vi "Calibrate.vi"(8 "error in (no error)":errorcluster, 11 "KUKA youBot arm motor_EtherCAT in":refnum<class "NI_Robotics_KUKA youBot Arm Motor_EtherCAT.lvclass">) -> (0 "error out":errorcluster, 3 "KUKA youBot arm motor_EtherCAT out":refnum<class "NI_Robotics_KUKA youBot Arm Motor_EtherCAT.lvclass">)   [LabVIEW 2017, in "NI_Robotics_KUKA youBot Host.lvlib" / "NI_Robotics_KUKA youBot Arm Motor_EtherCAT.lvclass"]
uses:
  <vilib>/robotics/KUKA youBot/Motor/Arm Motor EtherCAT/NI_Robotics_KUKA youBot Arm Motor_EtherCAT.lvclass
  <vilib>/robotics/KUKA youBot/Motor/Arm Motor EtherCAT/NI_Robotics_KUKA youBot Arm Motor_EtherCAT.lvclass/NI_Robotics_KUKA youBot Arm Motor_EtherCAT.ctl
  <vilib>/robotics/KUKA youBot/EtherCAT/EtherCAT Command.ctl
  <vilib>/robotics/KUKA youBot/EtherCAT/CmdCtrls/Param Cmd.ctl
  <vilib>/Platform/TimedLoop/XDataNode/timing_clust.ctl
  <vilib>/Platform/TimedLoop/XDataNode/nitl_modes.ctl
  <vilib>/Platform/TimedLoop/XDataNode/wakeup.ctl
  <vilib>/Platform/TimedLoop/XDataNode/XDataNode.xnode
  <vilib>/robotics/KUKA youBot/NI_Robotics_KUKA youBot Host.lvlib
  <vilib>/Platform/TimedLoop/XDataNode/XDNodeRunTimeDep.lvlib
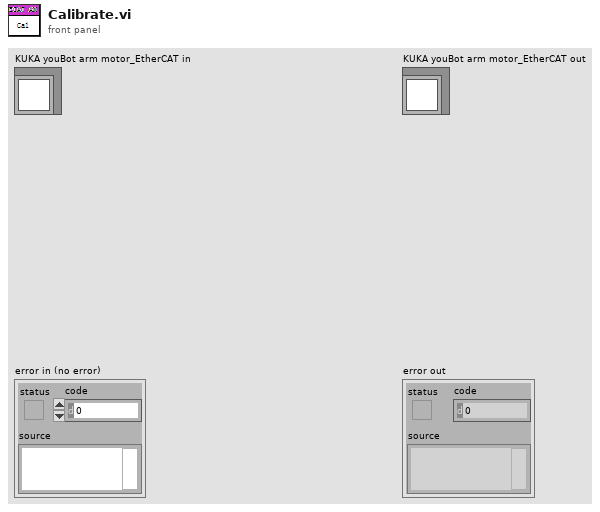
[diagram p1: front panel]
types:
  T1 = typedef "NI_Robotics_KUKA youBot Host.lvlib/EtherCAT Command.ctl" = cluster{"Module":u8, "Cmd":T2, "Type":u8, "Bank":u8, "Val":u32}
  T2 = typedef "NI_Robotics_KUKA youBot Host.lvlib/Param Cmd.ctl" = u8
  T3 = typedef "XDNodeRunTimeDep.lvlib/timing_clust.ctl" = cluster{"Expected End [f-1]":u64, "Actual End [f-1]":u64, "Finished Late? [f-1]":bool, "Expected End [i-1]":u64, "Actual End [i-1]":u64, "Finished Late? [i-1]":bool, "Expected Start [i]":u64, "Actual Start [i]":u64, "Expected Start [f]":u64, "Actual Start [f]":u64, "Source Name":string, "Structure Name":string, "Period":i64, "Deadline":i64, "Offset":i64, "Start":i64, "Priority":i32, "Timeout":i32, "Mode":T4, "Wakeup Reason":T5, "Error":errorcluster, "Source Type":string, "Secondary Source Type":string, "Global End Time":u64, "Global Start Time":u64, "Frame Duration":u64, "Iteration Duration":u64, "Assigned CPU":i32, "I/O Scan Engine Mode":u32}
  T4 = typedef "XDNodeRunTimeDep.lvlib/nitl_modes.ctl" = enum32{"No Change", "Process missed periods, maintain original phase", "Discard missed periods, maintain original phase", "Process missed periods, ignore original phase", "Discard missed periods, ignore original phase"}
  T5 = typedef "XDNodeRunTimeDep.lvlib/wakeup.ctl" = enum32{"Normal", "Aborted", "Asynchronous wakeup", "Timing source error", "Timed loop error", "Timeout"}
  T6 = typedef "NI_Robotics_KUKA youBot Host.lvlib/Mater Handler.ctl" = i32
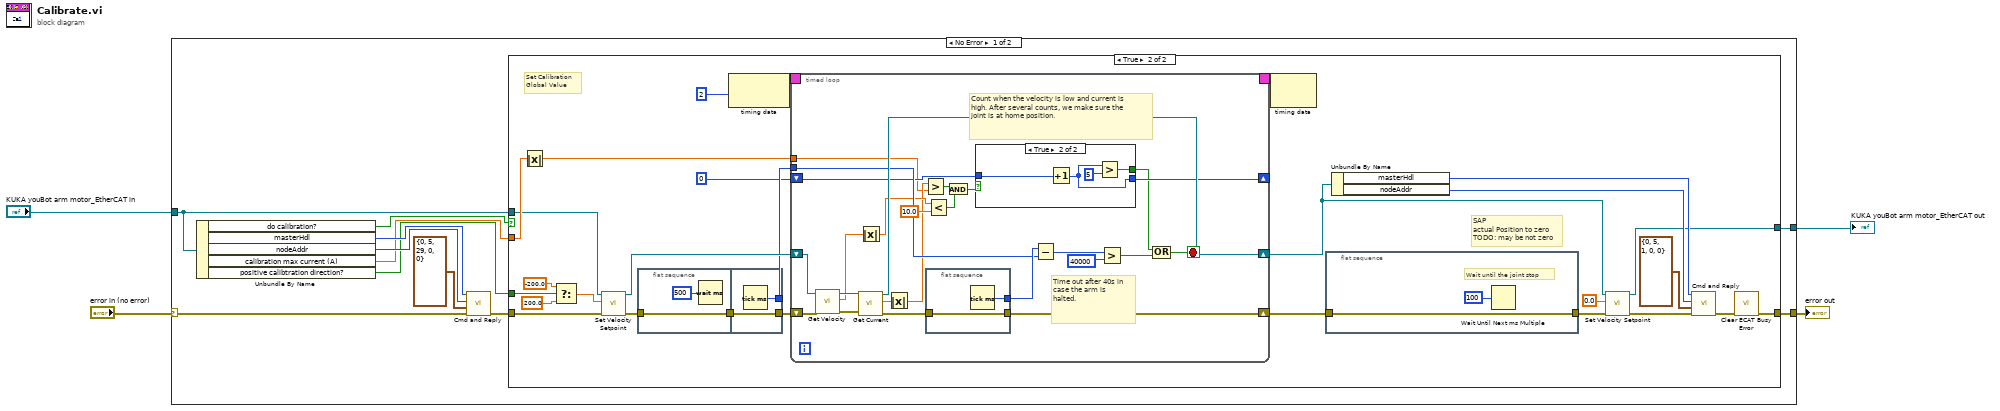
[diagram p0: block diagram]
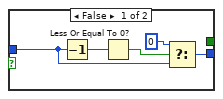
[diagram p3: hidden frame]
diagram:
  n1 = case shown="No Error" "error in (no error)" {
    selector: "error in (no error)" -> [w6 w95]
    tunnel: "KUKA youBot arm motor_EtherCAT in" -> [w7 w94]
    tunnel: [w10 w95] -> w2
    tunnel: [w9 w94] -> w1
    frame No Error {
      n2 = Unbundle By Name(w7) -> ("do calibration?"=w8:bool, "masterHdl"=w15:T6, "nodeAddr"=w14:u16, "calibration max current (A)"=w11:dbl, "positive calibtration direction?"=w12:bool)
      n3 = call <vilib>:"Cmd and Reply.vi"("error in (no error)"=w6, "EtherCAT command"=T1 {"Module"=0, "Cmd"=5, "Type"=29, "Bank"=0, "Val"=0} ("EtherCAT Command"), "nodeAddr in"=w14, "masterHdl in"=w15) -> ("error out"=w5:errorcluster)  [unwired: 3 in, 4 out]
      n4 = case shown="True" w8 {
        tunnel: w12 -> [_ w45]
        tunnel: w7 -> [w16 w26]
        tunnel: w5 -> [w17 w40]
        tunnel: w11 -> [_ w38]
        tunnel: [w17 w19] -> w10
        tunnel: [w16 w22] -> w9
        frame False {
        }
        frame True {
          # "Set Calibration\nGlobal Value"
          # "SAP\nactual Position to zero\nTODO: may be not zero"
          n5 = Absolute Value(x=w38) -> (abs(x)=w37:dbl)
          n6 = Select(t=-200.0, s=w45, f=200.0) -> (s? t:f=w31:dbl)
          n7 = call-dynamic "Set Velocity Setpoint.vi"("error in (no error)"=w40, "CCW velocity (rpm)"=w31, "KUKA youBot arm motor_EtherCAT in"=w26) -> ("error out"=w30:errorcluster, "KUKA youBot arm motor_EtherCAT out"=w39:refnum<class "NI_Robotics_KUKA youBot Arm Motor_EtherCAT.lvclass">)  [unwired: 7 in]
          n8 = flat-sequence {
            tunnel: w30 -> [w47]
            tunnel: [w47] -> w18
            tunnel: [w49] -> w29
            tunnel: [w48] -> w28
            tunnel: w18 -> [w49]
            frame #0 {
              n9 = Wait (ms)(milliseconds to wait=u32 500) -> ()  [unwired: 1 out]
            }
            frame #1 {
              n10 = Tick Count (ms)() -> (millisecond timer value=w48:u32)
            }
          }
          n11 = node-c288(i64 2 ("Period")) -> (w42:T3)
          n12 = timed-loop {
            timing: w42 -> [_]
            timing-out: [_] -> w41
            shift-right: [w76] -> w33
            shift-left: w39 -> [w61]
            tunnel: w37 -> [w52]
            shift-right: [w73] -> w36
            shift-left: w29 -> [w63]
            tunnel: w28 -> [w71]
            shift-right: [w66] -> _
            shift-left: 0 -> [w67]
            stop <- w74 stop-if-true
            # "Time out after 40s in case the arm is halted."
            # "Count when the velocity is low and current is high. After several counts, we make sure the joint is at home position."
            n13 = call-dynamic "Get Velocity.vi"("error in (no error)"=w63, "KUKA youBot Arm Motor_EtherCAT in"=w61) -> ("error out"=w62:errorcluster, "CCW velocity (rpm)"=w59:dbl, "KUKA youBot Arm Motor_EtherCAT out"=w60:refnum<class "NI_Robotics_KUKA youBot Arm Motor_EtherCAT.lvclass">)  [unwired: 7 in]
            n14 = call-dynamic "Get Current.vi"("error in (no error)"=w62, "KUKA youBot arm motor_EtherCAT in"=w60) -> ("error out"=w64:errorcluster, "current (A)"=w75:dbl, "KUKA youBot arm motor_EtherCAT out"=w76:refnum<class "NI_Robotics_KUKA youBot Arm Motor_EtherCAT.lvclass">)  [unwired: 7 in]
            n15 = Absolute Value(x=w59) -> (abs(x)=w54:dbl)
            n16 = Absolute Value(x=w75) -> (abs(x)=w53:dbl)
            n17 = Greater?(x=w53, y=w52) -> (0:w57:bool)
            n18 = flat-sequence {
              tunnel: w64 -> [w87]
              tunnel: [w87] -> w73
              tunnel: [w86] -> w72
              frame #0 {
                n19 = Tick Count (ms)() -> (millisecond timer value=w86:u32)
              }
            }
            n20 = Less?(x=w54, y=10.0) -> (x < y?=w56:bool)
            n21 = And(x=w57, y=w56) -> (x .and. y?=w55:bool)
            n22 = case shown="True" w55 {
              tunnel: w67 -> [w79 w85]
              tunnel: [w77 w84] -> w66
              tunnel: [_ w82] -> w65
              frame False {
                n23 = Decrement(x=w79) -> (x-1=w81:i32)
                n24 = Less Or Equal To 0?(x=w81) -> (x <= 0?=w80:bool)
                n25 = Select(t=0, s=w80, f=w79) -> (s? t:f=w77:i32)
              }
              frame True {
                n26 = Increment(x=w85) -> (x+1=w84:i32)
                n27 = Greater?(x=w84, y=5) -> (0:w82:bool)
              }
            }
            n28 = Subtract(x=w72, y=w71) -> (x-y=w70:u32)
            n29 = Greater?(x=w70, y=u32 40000) -> (0:w68:bool)
            n30 = Compound Arithmetic op=OR(w65, w68) -> (w74:bool)
          }
          n31 = node-c288(w41) -> ()  [unwired: 1 out]
          n32 = flat-sequence {
            tunnel: w36 -> [w50]
            tunnel: [w50] -> w34
            frame #0 {
              # "Wait until the joint stop"
              n33 = Wait Until Next ms Multiple(millisecond multiple=u32 100) -> ()  [unwired: 1 out]
            }
          }
          n34 = Unbundle By Name(w33) -> ("masterHdl"=w24:T6, "nodeAddr"=w23:u16)
          n35 = call-dynamic "Set Velocity Setpoint.vi"("error in (no error)"=w34, "CCW velocity (rpm)"=0.0 ("CCW Velocity (rad/s)"), "KUKA youBot arm motor_EtherCAT in"=w33) -> ("error out"=w21:errorcluster, "KUKA youBot arm motor_EtherCAT out"=w22:refnum<class "NI_Robotics_KUKA youBot Arm Motor_EtherCAT.lvclass">)  [unwired: 7 in]
          n36 = call <vilib>:"Cmd and Reply.vi"("error in (no error)"=w21, "EtherCAT command"=T1 {"Module"=0, "Cmd"=5, "Type"=1, "Bank"=0, "Val"=0} ("EtherCAT Command"), "nodeAddr in"=w23, "masterHdl in"=w24) -> ("error out"=w20:errorcluster)  [unwired: 3 in, 4 out]
          n37 = call <vilib>:"Clear ECAT Busy Error.vi"("error in (no error)"=w20) -> ("error out"=w19:errorcluster)  [unwired: 10 in]
        }
      }
    }
    frame Error {
    }
  }
  "error out" <- w2
  "KUKA youBot arm motor_EtherCAT out" <- w1
